vi "Configure Units.vi"(0 "VISA resource name":refnum<visa-resource-name>, 1 "Temperature Units (0: Celsius)":u16(ring) items=["Celsius", "Fahrenheit", "Kelvin"], 2 "DC Volts Units (0: Volts)":u16(ring) items=["Volts", "dB", "dBm"], 3 "AC Volts Units (0: Volts)":u16(ring) items=["Volts", "dB", "dBm"], 5 "error in (no error)":errorcluster, 6 "DC Reference Voltage (1.00000 V)":dbl=1.0 format="%_6g", 8 "DC Reference Impedance (75.00000 Ohm)":dbl=75.0 format="%_6g", 10 "AC Reference Voltage (1.00000 V)":dbl=1.0 format="%_6g", 12 "AC Reference Impedance (75.00000 Ohm)":dbl=75.0 format="%_6g") -> (14 "VISA resource name out":refnum<visa-resource-name>, 19 "error out":errorcluster)   [LabVIEW 2009, in "Keithley 2000.lvlib"]
doc: "This VI configures the units of various measurements on the instrument."
uses:
  <instrlib>/Keithley 2000/Keithley 2000.lvlib
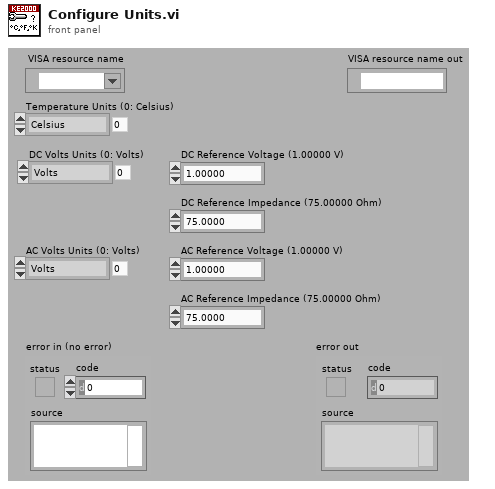
[diagram p1: front panel]
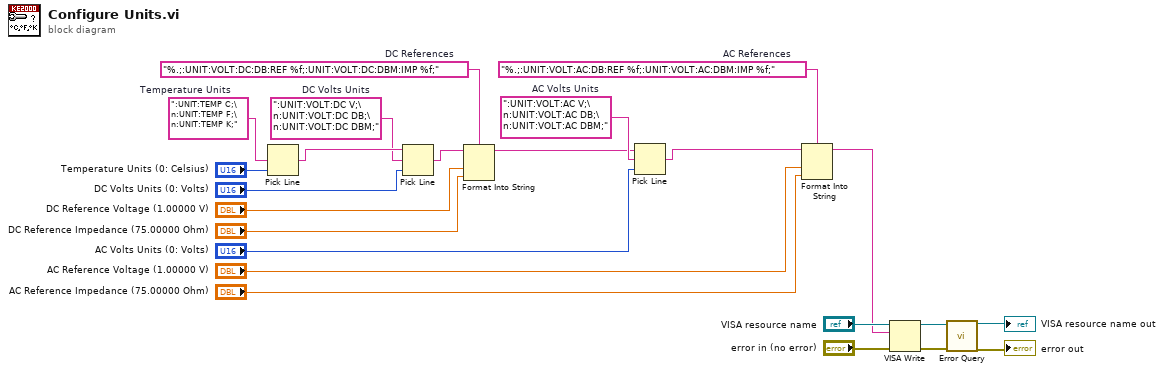
[diagram p0: block diagram]
diagram:
  w10 = "%.;:UNIT:VOLT:AC:DB:REF %f;:UNIT:VOLT:AC:DBM:IMP %f;"  # AC References
  w11 = "%.;:UNIT:VOLT:DC:DB:REF %f;:UNIT:VOLT:DC:DBM:IMP %f;"  # DC References
  w17 = ":UNIT:TEMP C;\n:UNIT:TEMP F;\n:UNIT:TEMP K;"  # Temperature Units
  w13 = ":UNIT:VOLT:AC V;\n:UNIT:VOLT:AC DB;\n:UNIT:VOLT:AC DBM;"  # AC Volts Units
  w14 = ":UNIT:VOLT:DC V;\n:UNIT:VOLT:DC DB;\n:UNIT:VOLT:DC DBM;"  # DC Volts Units
  n1 = Pick Line(multi-line string=w17, line index="Temperature Units (0: Celsius)") -> (output string=w15:string)  [unwired: 1 in]
  n2 = Pick Line(string ("")=w15, multi-line string=w14, line index="DC Volts Units (0: Volts)") -> (output string=w9:string)
  n3 = Format Into String(format string=w11, initial string=w9, "DC Reference Voltage (1.00000 V)", "DC Reference Impedance (75.00000 Ohm)") -> (resulting string=w5:string)  [unwired: 1 in, 1 out]
  n4 = Pick Line(string ("")=w5, multi-line string=w13, line index="AC Volts Units (0: Volts)") -> (output string=w6:string)
  n5 = Format Into String(format string=w10, initial string=w6, "AC Reference Voltage (1.00000 V)", "AC Reference Impedance (75.00000 Ohm)") -> (resulting string=w1:string)  [unwired: 1 in, 1 out]
  n6 = VISA Write(VISA resource name="VISA resource name", write buffer=w1, error in (no error)="error in (no error)") -> (VISA resource name out=w19:refnum<visa-resource-name>, error out=w18:errorcluster)  [unwired: 1 out]
  n7 = call <instrlib>:"Error Query.vi"("VISA resource name"=w19, "error in (no error)"=w18) -> ("VISA resource name out"=→"VISA resource name out":refnum<visa-resource-name>, "error out"=→"error out":errorcluster)  [unwired: 14 in, 2 out]
